vi "rtout_setTriggerConfig.vi"(0 "connection ID":refnum<k5>, 1 "axis":i32, 2 "higher":i32, 3 "lower":i32, 4 "epsilon":i32, 5 "error in":errorcluster, 7 "polarity":i32) -> (14 "connection ID":refnum<k5>, 15 "axis_out":i32, 19 "error out":errorcluster)   [LabVIEW 2016, in "AMC_VIs.lvlib"]
doc: "Control the real time output trigger config"
uses:
  AMC_VIs.lvlib
panel:
  out "params_cluster":T1
  in  "Params_cluster":T2
  in  "results_cluster":cluster{"errNo":i32}
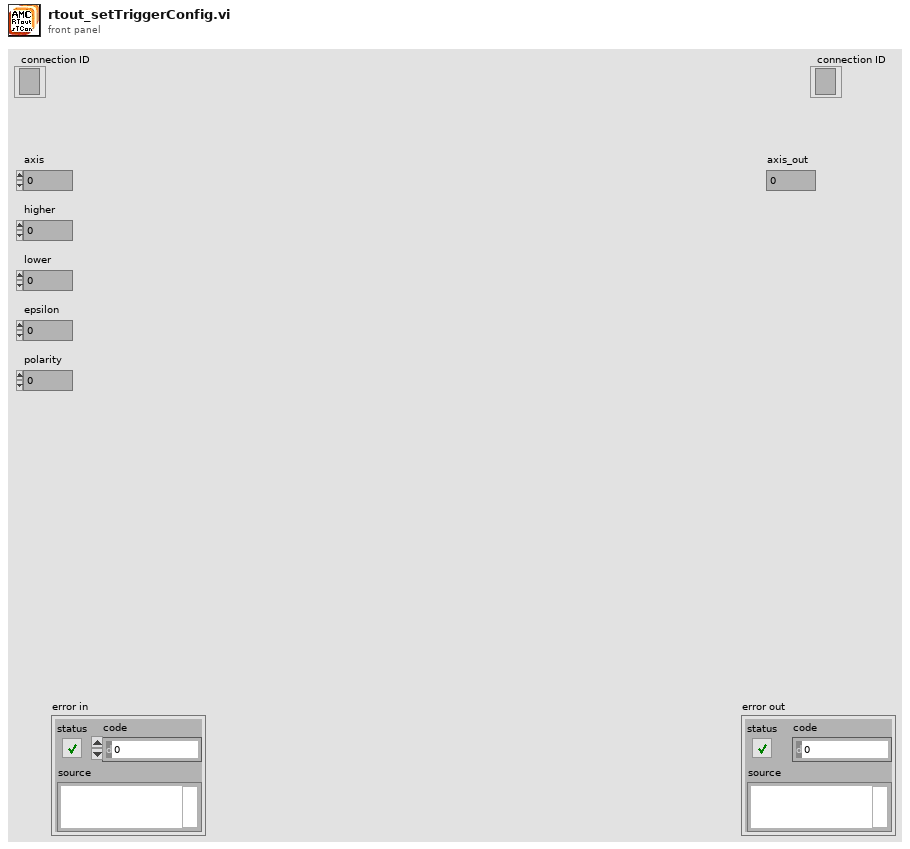
[diagram p1: front panel]
types:
  T1 = cluster{"axis":i32, "higher":i32, "lower":i32, "epsilon":i32, "polarity":i32}
  T2 = cluster{"integer":i32, "integer":i32, "integer":i32, "integer":i32, "integer":i32}
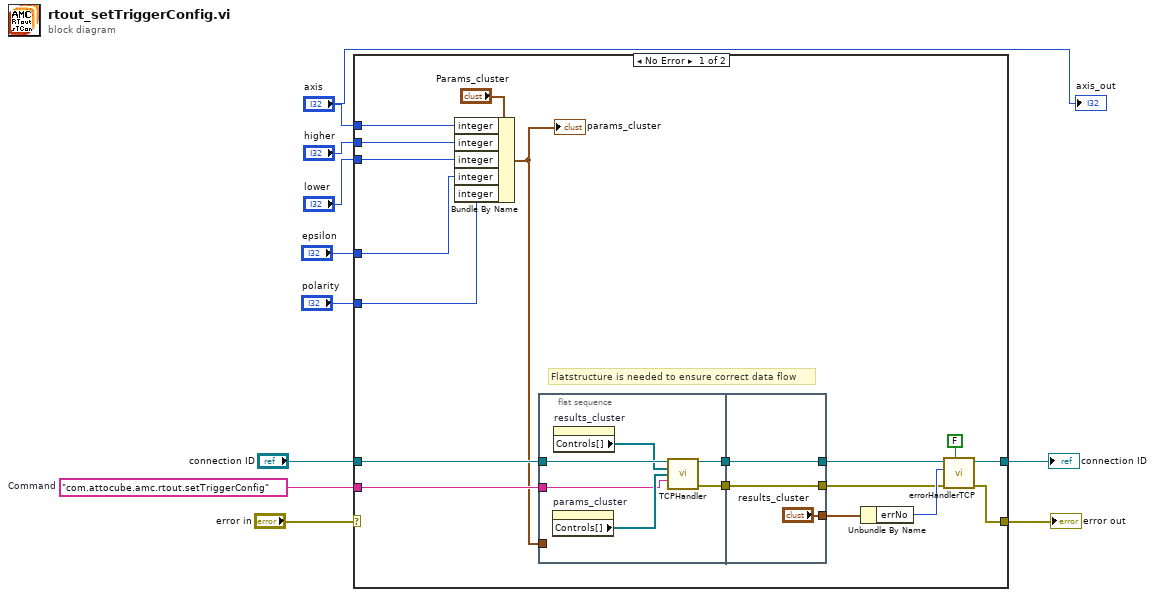
[diagram p0: block diagram]
diagram:
  w6 = "com.attocube.amc.rtout.setTriggerConfig"  # Command
  n1 = case shown="No Error" "error in" {
    selector: "error in" -> [_ w39]
    tunnel: [w26 w39] -> w10
    tunnel: [w28 w38] -> w9
    tunnel: "connection ID" -> [w25 w38]
    tunnel: w6 -> [w19 _]
    tunnel: "axis" -> [w15 _]
    tunnel: "higher" -> [w14 _]
    tunnel: "lower" -> [w13 _]
    tunnel: "epsilon" -> [w12 _]
    tunnel: "polarity" -> [w11 _]
    frame No Error {
      # "Flatstructure is needed to ensure correct data flow"
      n2 = Bundle By Name(cluster="Params_cluster", "integer"=w15, "integer"=w14, "integer"=w13, "integer"=w12, "integer"=w11) -> (w16:T2)
      "params_cluster" <- w16
      n3 = flat-sequence {
        tunnel: [w33] -> w21
        tunnel: w25 -> [w34]
        tunnel: w19 -> [w30]
        tunnel: [w29] -> w17
        tunnel: w16 -> [_]
        tunnel: ["results_cluster"] -> w22
        tunnel: [w37] -> w24
        tunnel: w21 -> [w37]
        tunnel: [w35] -> w18
        tunnel: w17 -> [w35]
        frame #0 {
          n4 = property on="params_cluster" class="Clust (strict)"() -> ("Controls[]"=w31:refnum<vi>[])  [unwired: 2 in, 2 out]
          n5 = property on="results_cluster" class="Clust (strict)"() -> ("Controls[]"=w32:refnum<vi>[])  [unwired: 2 in, 2 out]
          n6 = call "TCPHandler.vi"("connection ID"=w34, "results_cluster"=w32, "params_cluster"=w31, "method"=w30) -> ("connection ID"=w33:refnum<k5>, "error"=w29:errorcluster)  [unwired: 8 in, 2 out]
        }
        frame #1 {
        }
      }
      n7 = Unbundle By Name(w22) -> ("errNo"=w23:i32)
      n8 = call "errorHandlerTCP.vi"("show popup"=FALSE, "error in"=w18, "error number"=w23, "connection ID"=w24) -> ("error out"=w26:errorcluster, "connection ID"=w28:refnum<k5>)  [unwired: 6 in]
    }
    frame Error {
    }
  }
  "error out" <- w10
  "connection ID" <- w9
  "axis_out" <- "axis"
